vi "Actor Core.vi"(8 "error in":errorcluster, 11 "MWWL Verification":refnum<class "MWWL Verification.lvclass">) -> (0 "error out":errorcluster, 3 "Actor out":refnum<class "Actor.lvclass">)   [LabVIEW 2018, in "MWWL Verification.lvlib" / "MWWL Verification.lvclass"]
doc: "The purpose of this program is to allow an operator to dynamically select a microwave radar water level or bridge clearance (Air Gap) sensor and validate the range measurements by comparing to a series of high precision laser range finders (acquired from Dimetix & Laser Technologies Inc.)."
uses:
  MWWL Verification.lvclass
  C:/Program Files (x86)/National Instruments/LabVIEW 2018/vi.lib/ActorFramework/Actor/Actor.lvclass
  <vilib>/ActorFramework/Actor/Actor.lvclass
  Type Defs/Menu Items.ctl
  Type Defs/DLS Status LEDs.ctl
  Range Controller Actor/Typedefs/Verifier Enum.ctl
  <vilib>/ActorFramework/Actor/Actor.lvclass/Actor.ctl
  <vilib>/ActorFramework/Message Enqueuer/Message Enqueuer.lvclass/Message Enqueuer.ctl
  MWWL Verification.lvclass/MWWL Verification.ctl
  <vilib>/ActorFramework/Message Enqueuer/Init from Existing Queue.vi
  <vilib>/ActorFramework/Message Enqueuer/Enqueue.vi
  <vilib>/ActorFramework/Stop Msg/Stop Msg.lvclass
  C:/Program Files (x86)/National Instruments/LabVIEW 2018/vi.lib/ActorFramework/Message/Message.lvclass
  MWWL Verification Messages/Abort Msg/Abort Msg.lvclass
  <vilib>/ActorFramework/Message Priority Queue/Priority Enqueue.vi
  Actor Monitor/Actor/Monitored Actor.lvclass
  <vilib>/ActorFramework/Message Enqueuer/Message Enqueuer.lvclass
  MWWL Verification Messages/Initialize Reference Range Controller Msg/Initialize Reference Range Controller Msg.lvclass
  MWWL Verification Messages/Disabled Property(Main Controls)_Initialize Msg/Disabled Property(Main Controls)_Initialize Msg.lvclass
  MWWL Verification Messages/Move Target Manually Msg/Move Target Manually Msg.lvclass
  MWWL Verification Messages/Manual or Auto Controller Msg/Manual or Auto Controller Msg.lvclass
  MWWL Verification Messages/Set Desired Range Msg/Set Desired Range Msg.lvclass
  MWWL Verification Messages/Mean Range Values from FP Indicators Msg/Mean Range Values from FP Indicators Msg.lvclass
  MWWL Verification Messages/Disabled Property(Main Controls)_Measure Msg/Disabled Property(Main Controls)_Measure Msg.lvclass
  MWWL Verification Messages/Create Data Entry for Log Msg/Create Data Entry for Log Msg.lvclass
  MWWL Verification Messages/Initialize Datalogger Msg/Initialize Datalogger Msg.lvclass
  MWWL Verification.lvlib
panel:
  in  "Verifier State":T1
  out "Time Series":T2(graph)
  in  "Reference Range Controls":cluster{"FWD":bool, "REV":bool}
  in  "Recording?":bool
  in  "Target Range":dbl(slide) min=0.0 max=30.0 step=0.001 scale=0.0..30.0 scale format="%#.2g"
  in  "Fault?":bool
  in  "Main Controls":T3
  out "Ranges":T5 {"ULS" format="%.3g"; "LASER D" format="%.3g"; "LASER C" format="%.3g"; "LASER B" format="%.3g"; "Microwave" format="%.3g"; "LASER A" format="%.3g"}
  in  "stop signal":bool
  out "Event Log":string
  in  "WebBrowser":refnum<k7>(container)
  # "RANGES (m)"
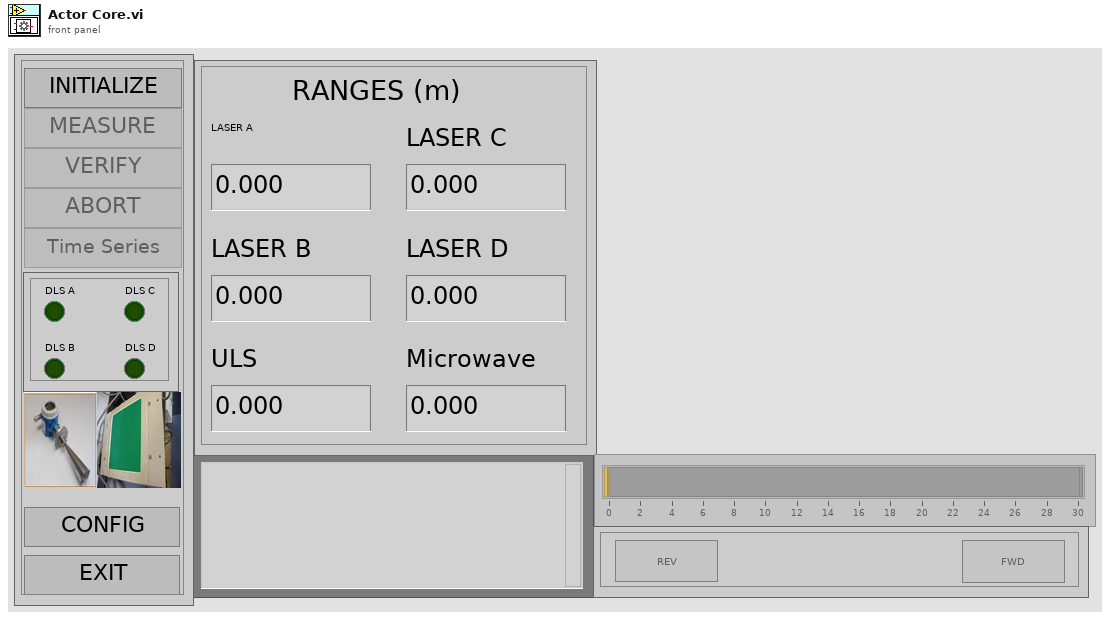
[diagram p1: front panel]
types:
  T1 = typedef "MWWL Verification.lvlib/Verifier Enum.ctl" = enum16{"Idle", "Begin Test", "Check Target Distance", "Move Target", "Save to Disk", "Check Desired Range"}
  T2 = cluster{"NewVal":dbl, "NewVal":dbl, "NewVal":dbl, "NewVal":dbl, "NewVal":dbl, "NewVal":dbl}
  T3 = typedef "MWWL Verification.lvlib/Menu Items.ctl" = cluster{"Initialize":bool, "Measure":bool, "Verify Button":bool, "Abort Button":bool, "Time Series":bool, "ULS Status":T4, "Config Button":bool, "Exit Button":bool}
  T4 = typedef "MWWL Verification.lvlib/DLS Status LEDs.ctl" = cluster{"DLS A":bool, "DLS B":bool, "DLS C":bool, "DLS D":bool}
  T5 = cluster{"LASER A":dbl, "LASER B":dbl, "LASER C":dbl, "LASER D":dbl, "ULS":dbl, "Microwave":dbl}
  T6 = enum8{"Enabled", "Disabled", "Disabled and Grayed Out"}
  T7 = typedef "MWWL Verification.lvlib/ConfigSettings.ctl" = cluster{"Base Path":path, "DNL_Configuration Settings.Ports":cluster{"Ref. Range COM Port":refnum<visa-resource-name>, "MWWL COM Port":refnum<visa-resource-name>, "ULS COM Port":refnum<visa-resource-name>, "Laser A COM Port":refnum<visa-resource-name>, "Laser B COM Port":refnum<visa-resource-name>, "Laser C COM Port":refnum<visa-resource-name>, "Laser D COM Port":refnum<visa-resource-name>, "AirMar COM Port":refnum<visa-resource-name>}, "H3611i":bool}
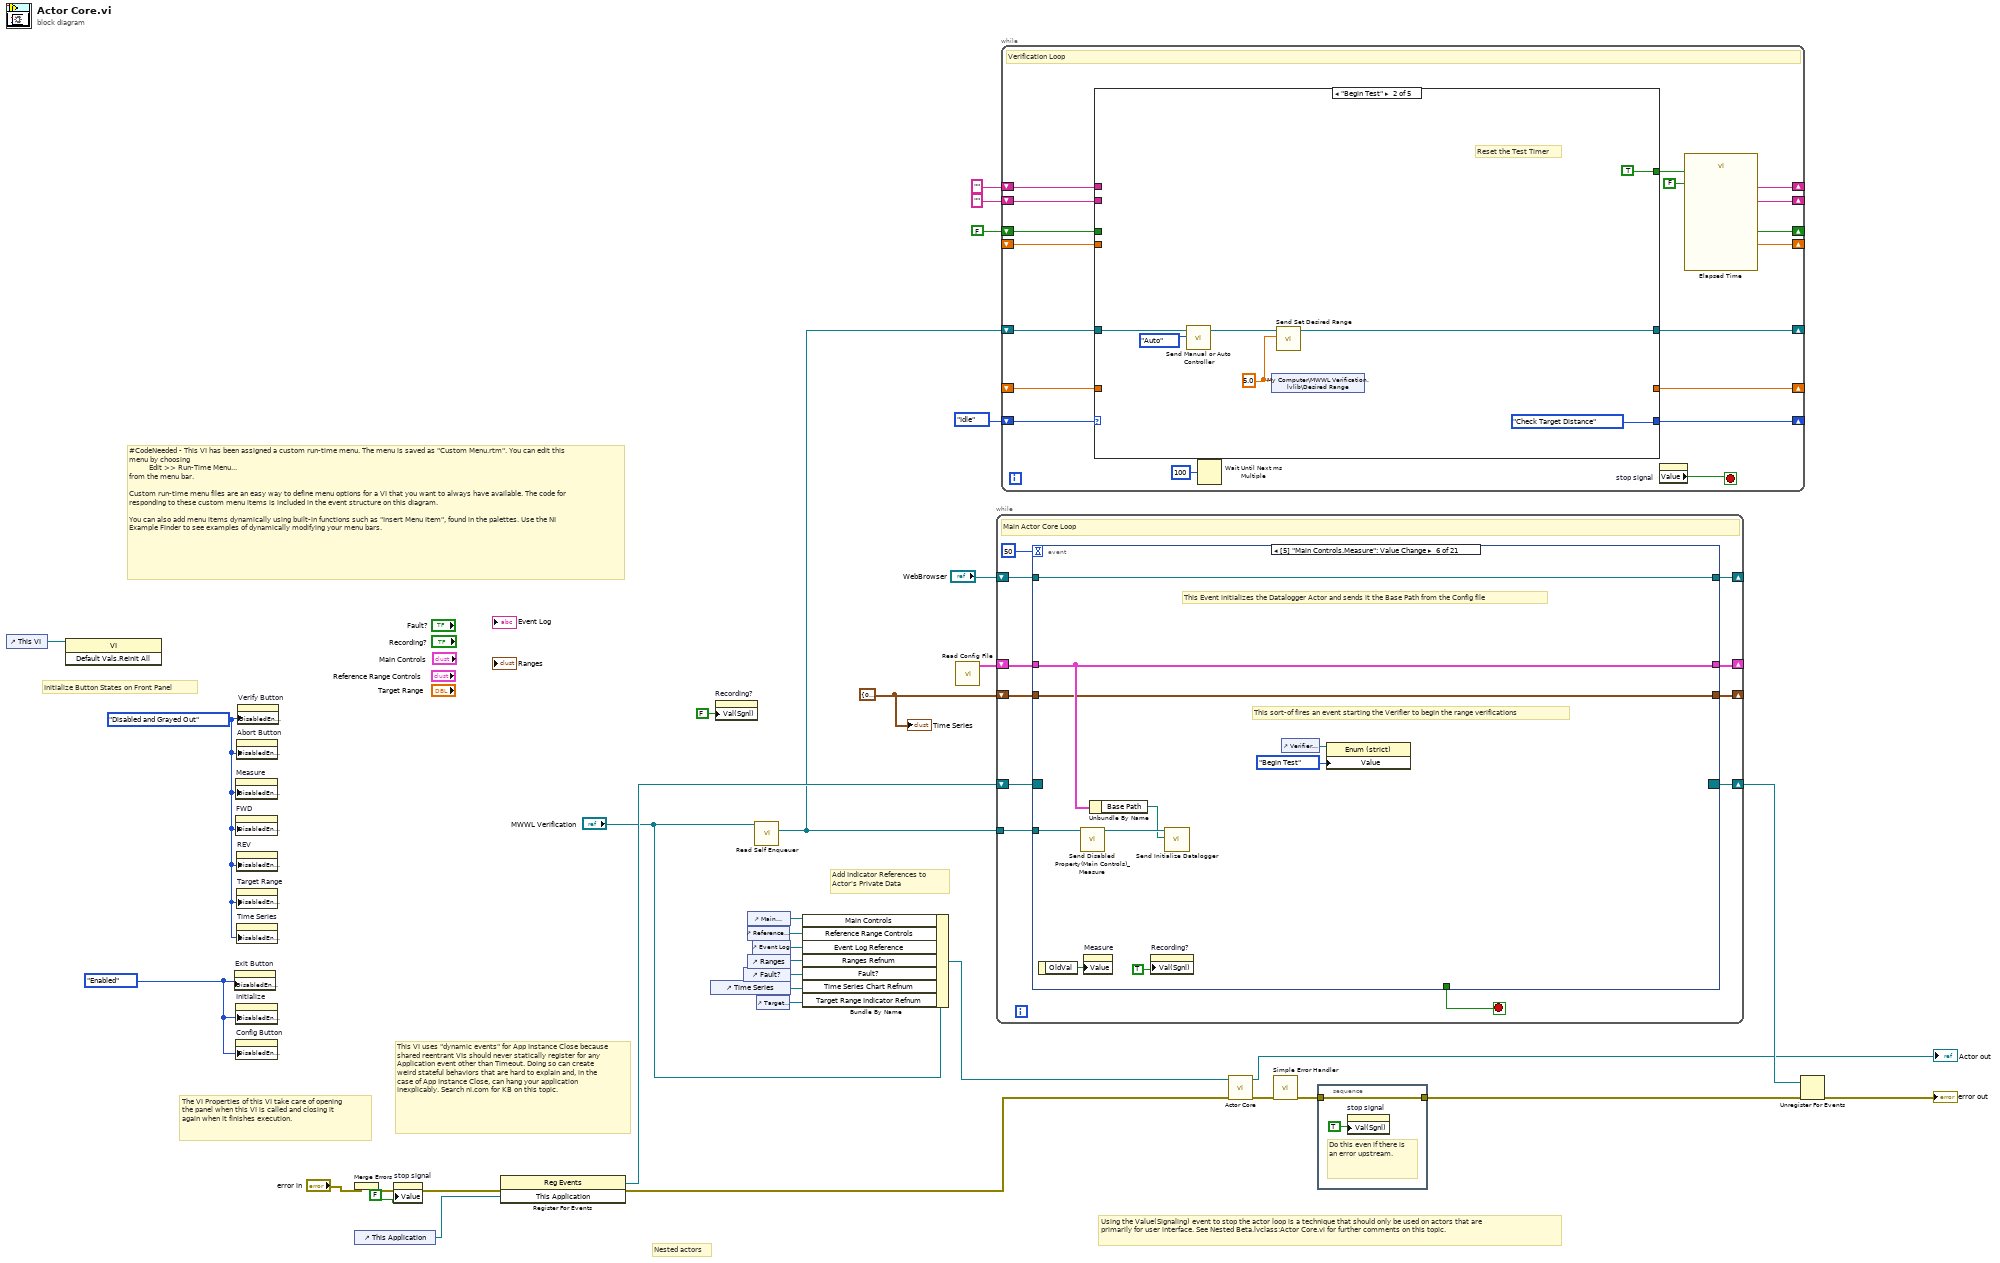
[diagram p0: block diagram]
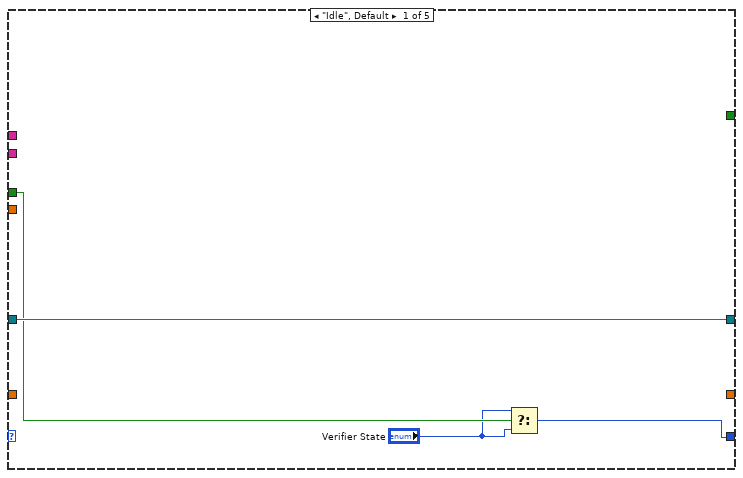
[diagram p2: hidden frame]
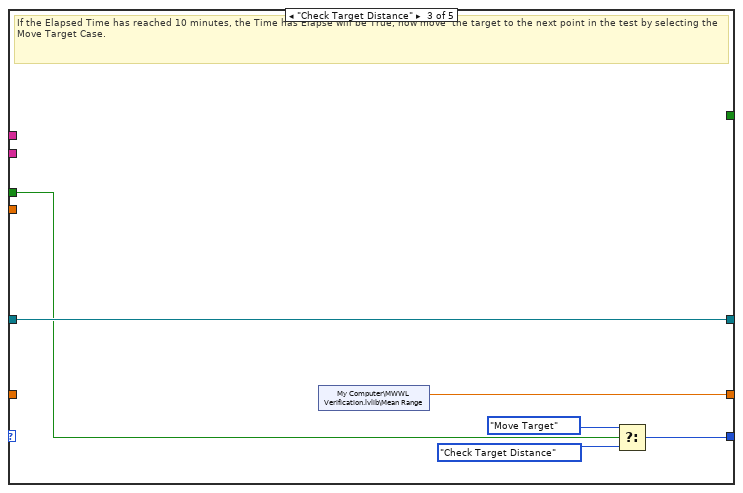
[diagram p3: hidden frame]
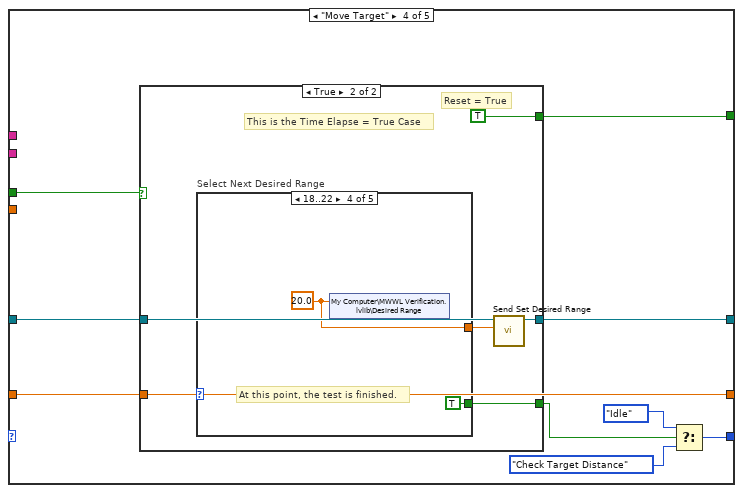
[diagram p4: hidden frame]
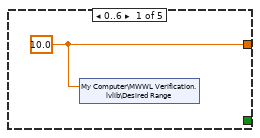
[diagram p6: hidden frame]
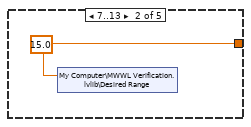
[diagram p7: hidden frame]
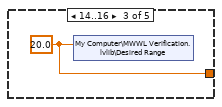
[diagram p8: hidden frame]
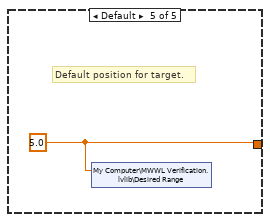
[diagram p9: hidden frame]
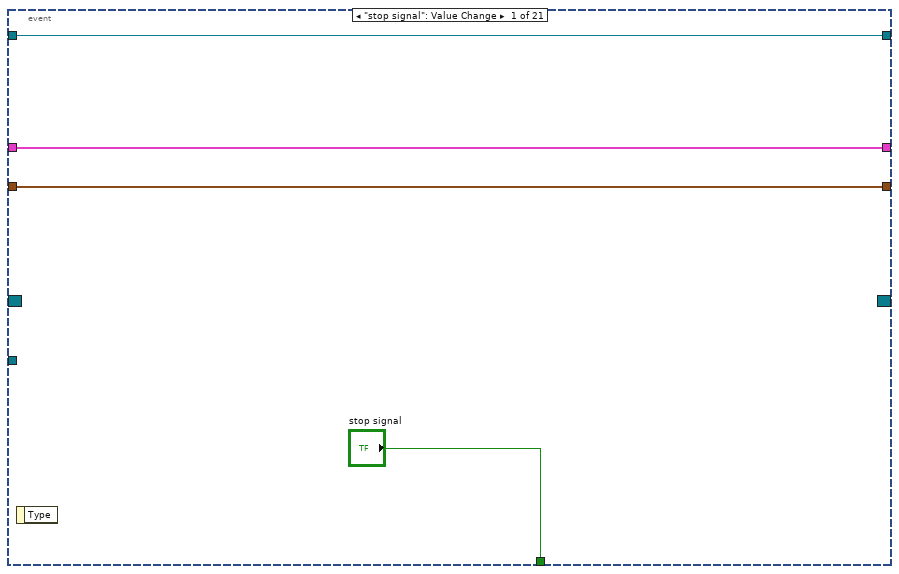
[diagram p11: hidden frame]
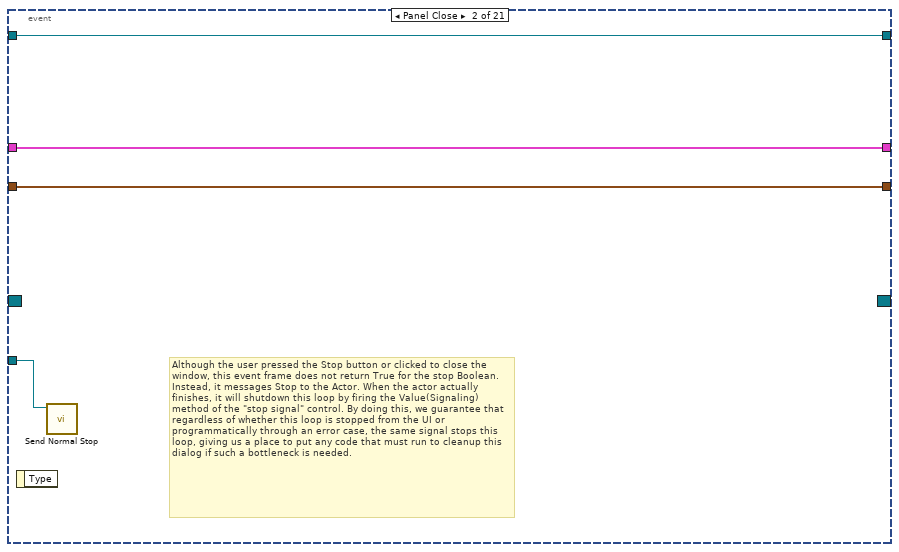
[diagram p12: hidden frame]
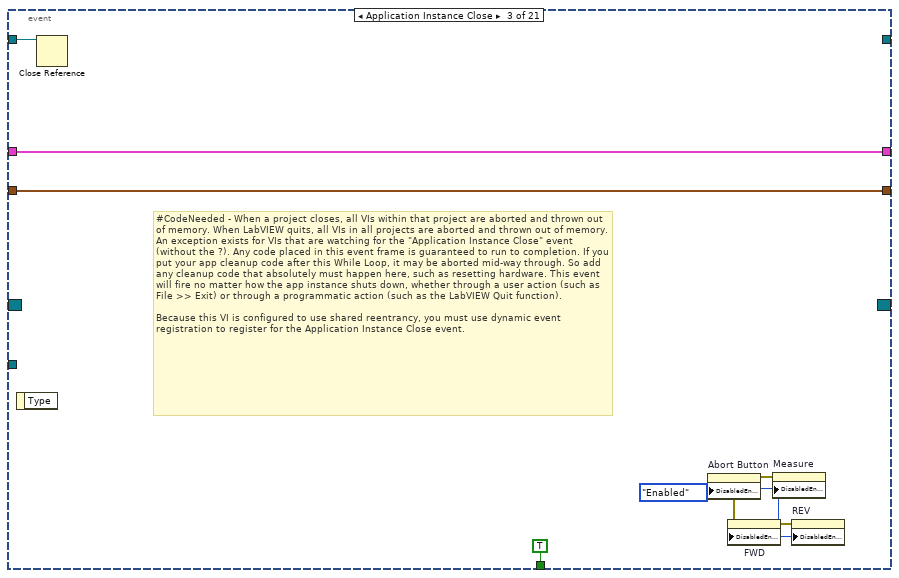
[diagram p13: hidden frame]
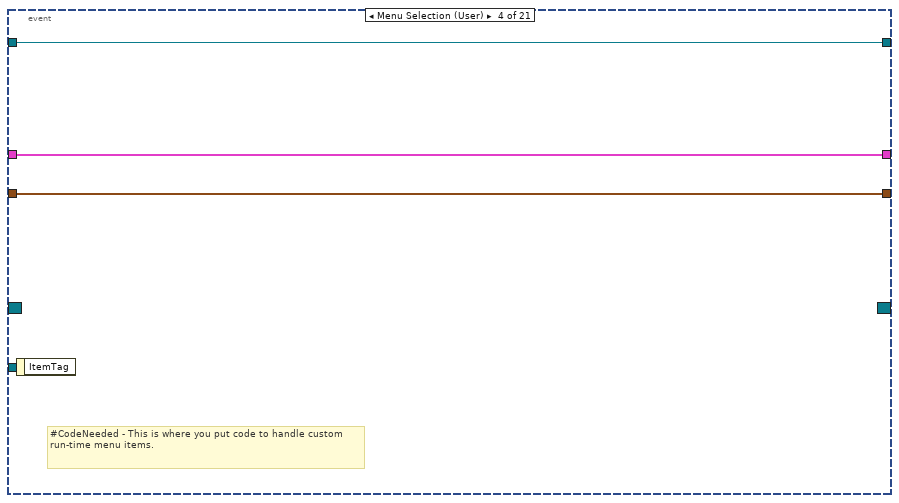
[diagram p14: hidden frame]
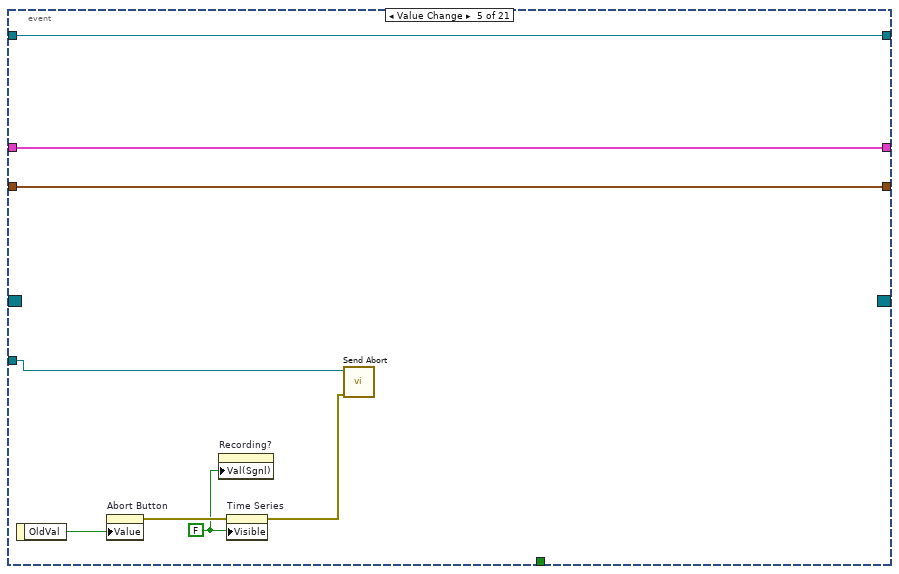
[diagram p15: hidden frame]
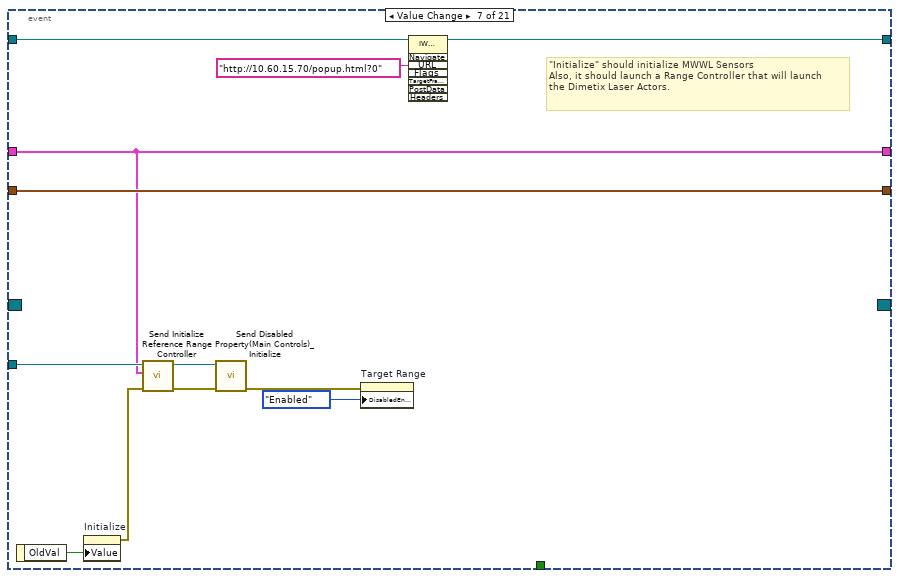
[diagram p16: hidden frame]
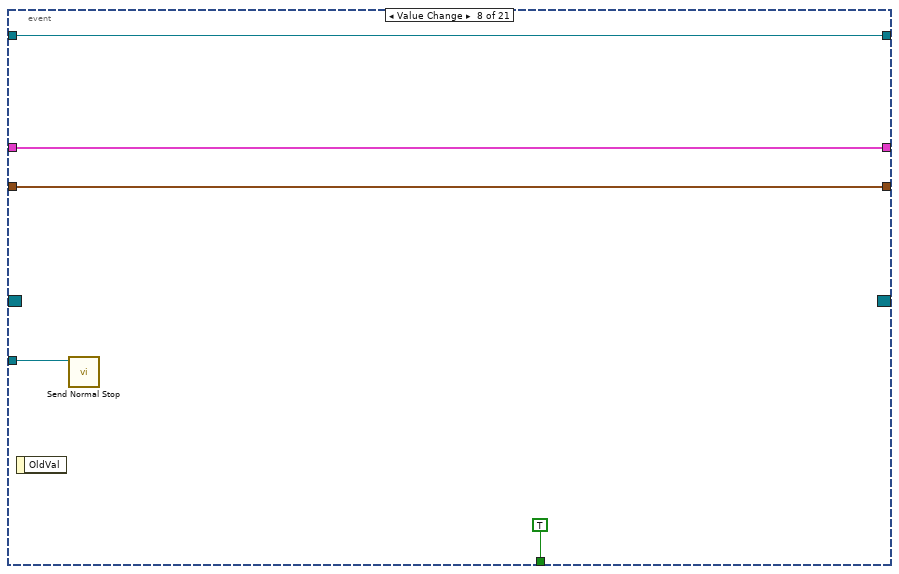
[diagram p17: hidden frame]
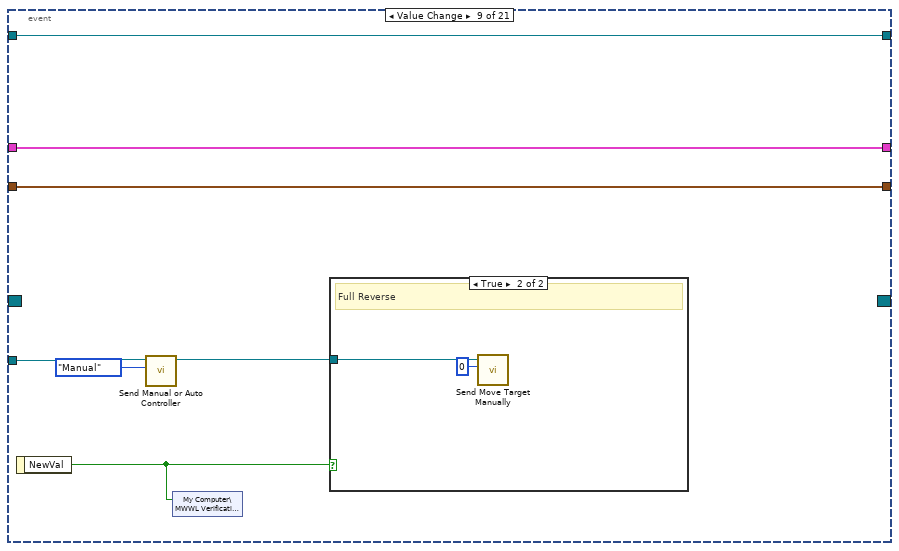
[diagram p18: hidden frame]
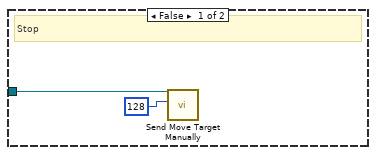
[diagram p19: hidden frame]
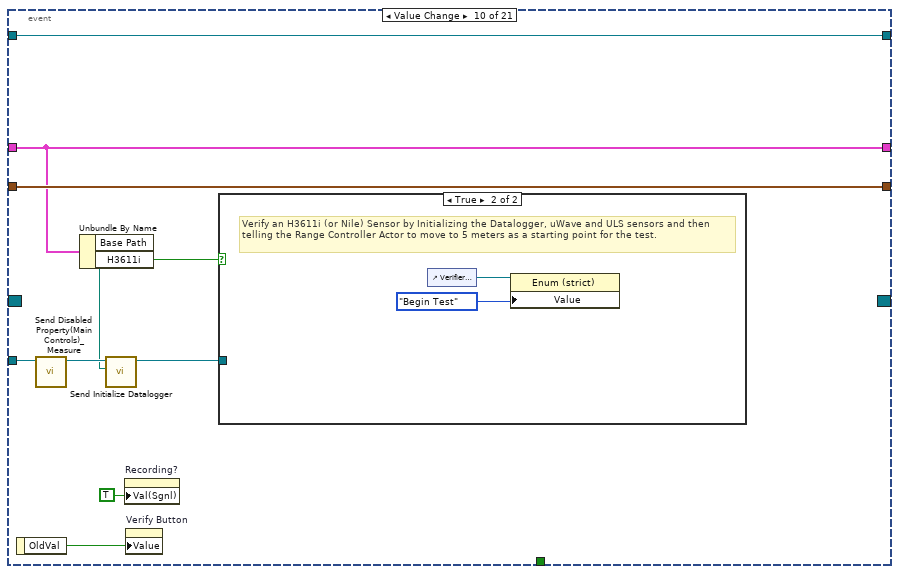
[diagram p20: hidden frame]
diagram:
  w9 = T5 {"LASER A"=0.0, "LASER B"=0.0, "LASER C"=0.0, "LASER D"=0.0, "ULS"=0.0, "Microwave"=0.0} ("Ranges")
  w12 = T6."Disabled and Grayed Out" ("Disabled")
  w11 = T6."Enabled" ("Disabled")
  # "Initialize Button States on Front Panel"
  # "Add Indicator References to \nActor's Private Data"
  # "Nested actors"
  # "#CodeNeeded - This VI has been assigned a custom run-time menu. The menu is saved as \"Custom Menu.rtm\". You can edit this menu by choosing \n          Edit >> Run-Time Menu...\nfrom the menu bar.\n\nCustom run-time menu files are an easy way to define menu options for a VI that you want to always have available. The code for responding to these custom menu items is included in the event structure on this diagram.\n\nYou can also add menu items dynamically using built-in functions such as \"Insert Menu Item\", found in the palettes. Use the NI Example Finder to see examples of dynamically modifying your menu bars."
  # "This VI uses \"dynamic events\" for App Instance Close because shared reentrant VIs should never statically register for any Application event other than Timeout. Doing so can create weird stateful behaviors that are hard to explain and, in the case of App Instance Close, can hang your application inexplicably. Search ni.com for KB on this topic."
  # "The VI Properties of this VI take care of opening the panel when this VI is called and closing it again when it finishes execution."
  # "Using the Value(Signaling) event to stop the actor loop is a technique that should only be used on actors that are primarily for user interface. See Nested Beta.lvclass:Actor Core.vi for further comments on this topic."
  n1 = control-ref of="This VI"() -> (w20:refnum<vi>)
  n2 = invoke class="VI" method="Default Vals.Reinit All"(reference=w20) -> ()  [unwired: 2 in, 3 out]
  n3 = property on="Exit Button" class="Bool"("DisabledEnum"=w11) -> ()  [unwired: 2 in, 2 out]
  n4 = property on="Measure" class="Bool (strict)"("DisabledEnum"=w12) -> ()  [unwired: 2 in, 2 out]
  n5 = property on="FWD" class="Bool (strict)"("DisabledEnum"=w12) -> ()  [unwired: 2 in, 2 out]
  n6 = property on="Initialize" class="Bool (strict)"("DisabledEnum"=w11) -> ()  [unwired: 2 in, 2 out]
  n7 = property on="Config Button" class="Bool (strict)"("DisabledEnum"=w11) -> ()  [unwired: 2 in, 2 out]
  n8 = property on="Abort Button" class="Bool (strict)"("DisabledEnum"=w12) -> ()  [unwired: 2 in, 2 out]
  n9 = property on="REV" class="Bool (strict)"("DisabledEnum"=w12) -> ()  [unwired: 2 in, 2 out]
  n10 = property on="Target Range" class="Slide (strict)"("DisabledEnum"=w12) -> ()  [unwired: 2 in, 2 out]
  n11 = property on="Time Series" class="Bool (strict)"("DisabledEnum"=w12) -> ()  [unwired: 2 in, 2 out]
  n12 = property on="Verify Button" class="Bool (strict)"("DisabledEnum"=w12) -> ()  [unwired: 2 in, 2 out]
  n13 = Merge Errors("error in") -> (w32:errorcluster)
  n14 = control-ref of="This Application"() -> (w3:refnum<vi>)
  n15 = property on="stop signal" class="Bool (strict)"(error in=w32, "Value"=FALSE ("stop")) -> (error out=w26:errorcluster)  [unwired: 1 in, 1 out]
  n16 = register-events(error in=w26, w3) -> (reference out=w29:refnum<event-registration>, error out=w23:errorcluster)  [unwired: 1 in]
  n17 = control-ref of="Time Series"() -> (w10:refnum<vi>)
  n18 = property on="Recording?" class="Bool (strict)"("Val(Sgnl)"=FALSE ("Value (Signaling)")) -> ()  [unwired: 2 in, 2 out]
  n19 = control-ref of="Fault?"() -> (w22:refnum<vi>)
  n20 = control-ref of="Reference Range Controls"() -> (w14:refnum<vi>)
  n21 = control-ref of="Main Controls"() -> (w16:refnum<vi>)
  n22 = control-ref of="Ranges"() -> (w21:refnum<vi>)
  n23 = control-ref of="Event Log"() -> (w34:refnum<vi>)
  n24 = call <vilib>:"Read Self Enqueuer.vi"("Actor"="MWWL Verification") -> ("Self Enqueuer"=w6:refnum<class "Message Enqueuer.lvclass">)  [unwired: 10 in]
  n25 = control-ref of="Target Range"() -> (w15:refnum<vi>)
  n26 = Bundle By Name(cluster="MWWL Verification", "Main Controls"=w16, "Reference Range Controls"=w14, "Event Log Reference"=w34, "Ranges Refnum"=w21, "Fault?"=w22, "Time Series Chart Refnum"=w10, "Target Range Indicator Refnum"=w15) -> (w19:refnum<class "MWWL Verification.lvclass">)
  n27 = call "Read Config File.vi"() -> ("Settings Out"=w25:T7)  [unwired: 10 in, 1 out]
  n28 = while {
    tunnel: w6 -> [w45]
    shift-right: [w42] -> w28
    shift-left: w29 -> [w43]
    shift-right: [w40] -> _
    shift-left: w25 -> [w41]
    shift-right: [w37] -> _
    shift-left: w9 -> [w36]
    shift-right: [w35] -> _
    shift-left: "WebBrowser" -> [w39]
    stop <- w44 stop-if-true
    # "Main Actor Core Loop"
    n29 = event shown="[5] \"Main Controls.Measure\": Value Change" {
      selector: w43 -> [_ _ _ _ _ _ _ _ _ _ _ _ _ _ _ _ _ _ _ _ _]
      dyn-events: [_ _ _ _ _ _ _ _ _ _ _ _ _ _ _ _ _ _ _ _ _] -> w42
      timeout: 50 -> [_ _ _ _ _ _ _ _ _ _ _ _ _ _ _ _ _ _ _ _ _]
      tunnel: w45 -> [_ w53 _ _ w71 w81 w91 w99 w105 w114 w126 w139 _ w153 _ w169 w187 w205 w223 w241 w252]
      tunnel: ["stop signal" _ TRUE ("stop signal") _ _ _ _ TRUE ("stop signal") _ _ _ _ _ _ _ _ _ _ _ _ _] -> w44
      tunnel: w41 -> [w48 w52 w61 w64 w72 w79 w83 w97 w106 w115 w129 w140 w146 w154 w162 w170 w188 w206 w224 w242 w253]
      tunnel: [w48 w52 w61 w64 w72 w79 w83 w97 w106 w115 w129 w140 w146 w154 w161 w170 w188 w206 w224 w242 w253] -> w40
      tunnel: w39 -> [w46 w50 w56 w62 w65 w75 w94 w95 w100 w118 w123 w134 w141 w149 w159 w164 w182 w200 w219 w236 w247]
      tunnel: w36 -> [w47 w51 w55 w63 w67 w76 w85 w96 w101 w119 w124 w135 w144 w150 w160 w167 w185 w203 w218 w238 w249]
      tunnel: [w47 w51 w55 w63 w67 w76 w85 w96 w101 w119 w124 w135 w144 w150 w160 w166 w183 w202 w220 w237 w248] -> w37
      tunnel: [w46 w50 _ w62 w65 w75 w84 w95 w100 w118 w123 w134 w141 w149 w159 w164 w182 w200 w219 w236 w247] -> w35
      event "stop signal": Value Change {
        n30 = event-data() -> ()  [unwired: 1 in, 1 out]
      }
      event Panel Close {
        # "Although the user pressed the Stop button or clicked to close the window, this event frame does not return True for the stop Boolean. Instead, it messages Stop to the Actor. When the actor actually finishes, it will shutdown this loop by firing the Value(Signaling) method of the \"stop signal\" control. By doing this, we guarantee that regardless of whether this loop is stopped from the UI or programmatically through an error case, the same signal stops this loop, giving us a place to put any code that must run to cleanup this dialog if such a bottleneck is needed."
        n31 = event-data() -> ()  [unwired: 1 in, 1 out]
        n32 = call <vilib>:"Send Normal Stop.vi"("Message Enqueuer"=w53) -> ()  [unwired: 10 in, 1 out]
      }
      event Application Instance Close {
        w58 = T6."Enabled" ("Disabled")
        # "#CodeNeeded - When a project closes, all VIs within that project are aborted and thrown out of memory. When LabVIEW quits, all VIs in all projects are aborted and thrown out of memory. An exception exists for VIs that are watching for the \"Application Instance Close\" event (without the ?). Any code placed in this event frame is guaranteed to run to completion. If you put your app cleanup code after this While Loop, it may be aborted mid-way through. So add any cleanup code that absolutely must happen here, such as resetting hardware. This event will fire no matter how the app instance shuts down, whether through a user action (such as File >> Exit) or through a programmatic action (such as the LabVIEW Quit function).\n\nBecause this VI is configured to use shared reentrancy, you must use dynamic event registration to register for the Application Instance Close event."
        n33 = event-data() -> ()  [unwired: 1 in, 1 out]
        n34 = Close Reference(reference=w56) -> ()  [unwired: 1 in, 1 out]
        n35 = property on="Abort Button" class="Bool (strict)"("DisabledEnum"=w58) -> (error out=w57:errorcluster)  [unwired: 2 in, 1 out]
        n36 = property on="Measure" class="Bool (strict)"(error in=w57, "DisabledEnum"=w58) -> (error out=w59:errorcluster)  [unwired: 1 in, 1 out]
        n37 = property on="FWD" class="Bool (strict)"(error in=w59, "DisabledEnum"=w58) -> (error out=w60:errorcluster)  [unwired: 1 in, 1 out]
        n38 = property on="REV" class="Bool (strict)"(error in=w60, "DisabledEnum"=w58) -> ()  [unwired: 1 in, 2 out]
      }
      event Menu Selection (User) {
        # "#CodeNeeded - This is where you put code to handle custom run-time menu items."
        n39 = event-data() -> ()  [unwired: 1 in, 1 out]
      }
      event Value Change {
        w66 = FALSE ("Visible")
        n40 = event-data() -> ("OldVal"=w70:bool)  [unwired: 1 in]
        n41 = property on="Abort Button" class="Bool (strict)"("Value"=w70) -> (error out=w69:errorcluster)  [unwired: 2 in, 1 out]
        n42 = property on="Recording?" class="Bool (strict)"("Val(Sgnl)"=w66) -> ()  [unwired: 2 in, 2 out]
        n43 = property on="Time Series" class="WFChart (strict)"(error in=w69, "Visible"=w66) -> (error out=w68:errorcluster)  [unwired: 1 in, 1 out]
        n44 = call "Send Abort.vi"("error in (no error)"=w68, "Message Enqueuer in"=w71) -> ()  [unwired: 8 in, 2 out]
      }
      event Value Change {
        # "This sort-of fires an event starting the Verifier to begin the range verifications"
        # "This Event initializes the Datalogger Actor and sends it the Base Path from the Config file"
        n45 = event-data() -> ("OldVal"=w82:bool)  [unwired: 1 in]
        n46 = call "Send Disabled Property(Main Controls)_Measure.vi"("Message Enqueuer in"=w81) -> ("Message Enqueuer out"=w80:refnum<class "Message Enqueuer.lvclass">)  [unwired: 9 in, 1 out]
        n47 = property on="Measure" class="Bool (strict)"("Value"=w82) -> ()  [unwired: 2 in, 2 out]
        n48 = Unbundle By Name(w79) -> ("Base Path"=w78:path)
        n49 = property on="Recording?" class="Bool (strict)"("Val(Sgnl)"=TRUE ("Value (Signaling)")) -> ()  [unwired: 2 in, 2 out]
        n50 = call "Send Initialize Datalogger.vi"("Base File Path"=w78, "Message Enqueuer in"=w80) -> ()  [unwired: 8 in, 2 out]
        n51 = control-ref of="Verifier State"() -> (w74:refnum<vi>)
        n52 = property class="Enum (strict)"(reference=w74, "Value"=Verifier_Enum."Begin Test" ("Verifier State")) -> ()  [unwired: 1 in, 2 out]
      }
      event Value Change {
        # "\"Initialize\" should initialize MWWL Sensors\nAlso, it should launch a Range Controller that will launch\nthe Dimetix Laser Actors."
        n53 = event-data() -> ("OldVal"=w89:bool)  [unwired: 1 in]
        n54 = property on="Initialize" class="Bool (strict)"("Value"=w89) -> (error out=w88:errorcluster)  [unwired: 2 in, 1 out]
        n55 = call "Send Initialize Reference Range Controller.vi"("error in (no error)"=w88, "Settings"=w83, "Message Enqueuer in"=w91) -> ("error out"=w90:errorcluster, "Message Enqueuer out"=w92:refnum<class "Message Enqueuer.lvclass">)  [unwired: 7 in]
        n56 = call "Send Disabled Property(Main Controls)_Initialize.vi"("error in (no error)"=w90, "Message Enqueuer in"=w92) -> ("error out"=w86:errorcluster)  [unwired: 8 in, 1 out]
        n57 = property on="Target Range" class="Slide (strict)"(error in=w86, "DisabledEnum"=T6."Enabled" ("Disabled")) -> ()  [unwired: 1 in, 2 out]
        n58 = invoke class="IWebBrowser2" method="Navigate"(reference=w94, "URL"="http://10.60.15.70/popup.html?0") -> (reference out=w84:refnum<k7>)  [unwired: 6 in, 7 out]
      }
      event Value Change {
        n59 = event-data() -> ()  [unwired: 1 in, 1 out]
        n60 = call <vilib>:"Send Normal Stop.vi"("Message Enqueuer"=w99) -> ()  [unwired: 10 in, 1 out]
      }
      event "Reference Range Controls.FWD": Value Change {
        n61 = event-data() -> ("NewVal"=w102:bool)  [unwired: 1 in]
        n62 = call "Send Manual or Auto Controller.vi"("Controller State"=enum16{"Manual", "Auto"}."Manual", "Message Enqueuer in"=w105) -> ("Message Enqueuer out"=w103:refnum<class "Message Enqueuer.lvclass">)  [unwired: 8 in, 1 out]
        n63 = shared-variable "My Computer\\MWWL Verification.lvlib\\FWD"(w102) -> ()  [unwired: 1 in, 1 out]
        n64 = case shown="True" w102 {
          tunnel: w103 -> [w107 w110]
          frame False {
            # "Stop"
            n65 = call "Send Move Target Manually.vi"("Target Speed & Direction"=i16 128, "Message Enqueuer in"=w107) -> ()  [unwired: 8 in, 2 out]
          }
          frame True {
            # "Full Reverse"
            n66 = call "Send Move Target Manually.vi"("Target Speed & Direction"=i16 0, "Message Enqueuer in"=w110) -> ()  [unwired: 8 in, 2 out]
          }
        }
      }
      event Value Change {
        n67 = event-data() -> ("OldVal"=w120:bool)  [unwired: 1 in]
        n68 = call "Send Disabled Property(Main Controls)_Measure.vi"("Message Enqueuer in"=w114) -> ("Message Enqueuer out"=w117:refnum<class "Message Enqueuer.lvclass">)  [unwired: 9 in, 1 out]
        n69 = Unbundle By Name(w115) -> ("Base Path"=w116:path, "H3611i"=w112:bool)
        n70 = call "Send Initialize Datalogger.vi"("Base File Path"=w116, "Message Enqueuer in"=w117) -> ("Message Enqueuer out"=w111:refnum<class "Message Enqueuer.lvclass">)  [unwired: 8 in, 1 out]
        n71 = property on="Recording?" class="Bool (strict)"("Val(Sgnl)"=TRUE ("Value (Signaling)")) -> ()  [unwired: 2 in, 2 out]
        n72 = property on="Verify Button" class="Bool (strict)"("Value"=w120) -> ()  [unwired: 2 in, 2 out]
        n73 = case shown="True" w112 {
          tunnel: w111 -> [_ _]
          frame False {
          }
          frame True {
            # "Verify an H3611i (or Nile) Sensor by Initializing the Datalogger, uWave and ULS sensors and then telling the Range Controller Actor to move to 5 meters as a starting point for the test."
            n74 = control-ref of="Verifier State"() -> (w122:refnum<vi>)
            n75 = property class="Enum (strict)"(reference=w122, "Value"=Verifier_Enum."Begin Test" ("Verifier State")) -> ()  [unwired: 1 in, 2 out]
          }
        }
      }
      event "Reference Range Controls.REV": Value Change {
        n76 = event-data() -> ("NewVal"=w125:bool)  [unwired: 1 in]
        n77 = shared-variable "My Computer\\MWWL Verification.lvlib\\REV"(w125) -> ()  [unwired: 1 in, 1 out]
        n78 = call "Send Manual or Auto Controller.vi"("Controller State"=enum16{"Manual", "Auto"}."Manual", "Message Enqueuer in"=w126) -> ("Message Enqueuer out"=w128:refnum<class "Message Enqueuer.lvclass">)  [unwired: 8 in, 1 out]
        n79 = case shown="True" w125 {
          tunnel: w128 -> [w130 w133]
          frame False {
            # "Stop"
            n80 = call "Send Move Target Manually.vi"("Target Speed & Direction"=i16 128, "Message Enqueuer in"=w130) -> ()  [unwired: 8 in, 2 out]
          }
          frame True {
            # "Full Reverse"
            n81 = call "Send Move Target Manually.vi"("Target Speed & Direction"=i16 255, "Message Enqueuer in"=w133) -> ()  [unwired: 8 in, 2 out]
          }
        }
      }
      event "Target Range": Value Change {
        n82 = event-data() -> ("NewVal"=w136:dbl)  [unwired: 1 in]
        n83 = call "Send Manual or Auto Controller.vi"("Controller State"=enum16{"Manual", "Auto"}."Auto", "Message Enqueuer in"=w139) -> ("Message Enqueuer out"=w137:refnum<class "Message Enqueuer.lvclass">)  [unwired: 8 in, 1 out]
        n84 = shared-variable "My Computer\\MWWL Verification.lvlib\\Desired Range"(w136) -> ()  [unwired: 1 in, 1 out]
        n85 = call "Send Set Desired Range.vi"("Desired Range"=w136, "Message Enqueuer in"=w137) -> ()  [unwired: 8 in, 2 out]
      }
      event Value Change {
        n86 = event-data() -> ("OldVal"=w145:bool)  [unwired: 1 in]
        n87 = property on="Time Series" class="Bool (strict)"("Value"=w145) -> ()  [unwired: 2 in, 2 out]
        n88 = control-ref of="Time Series"() -> (w148:refnum<vi>)
        n89 = property class="WFChart (strict)"(reference=w148) -> (reference out=w147:refnum<vi>, "Visible"=w142:bool)  [unwired: 1 in, 1 out]
        n90 = Not(x=w142) -> (.not. x?=w143:bool)
        n91 = property class="WFChart (strict)"(reference=w147, "Visible"=w143) -> ()  [unwired: 1 in, 2 out]
        n92 = property on="WebBrowser" class="AXCont"("Visible"=w142) -> ()  [unwired: 2 in, 2 out]
      }
      event Timeout {
        n93 = event-data() -> ()  [unwired: 1 in, 1 out]
        n94 = call "Send Mean Range Values from FP Indicators.vi"("Message Enqueuer in"=w153) -> ()  [unwired: 9 in, 2 out]
        n95 = control-ref of="FWD"() -> (w157:refnum<vi>)
        n96 = shared-variable "My Computer\\MWWL Verification.lvlib\\FWD"() -> (w158:bool)  [unwired: 1 in, 1 out]
        n97 = shared-variable "My Computer\\MWWL Verification.lvlib\\REV"() -> (w155:bool)  [unwired: 1 in, 1 out]
        n98 = control-ref of="REV"() -> (w156:refnum<vi>)
        n99 = control-ref of="Target Range"() -> (w152:refnum<vi>)
        n100 = shared-variable "My Computer\\MWWL Verification.lvlib\\Desired Range"() -> (w151:dbl)  [unwired: 1 in, 1 out]
        n101 = property class="Bool (strict)"(reference=w157, "Value"=w158) -> ()  [unwired: 1 in, 2 out]
        n102 = property class="Bool (strict)"(reference=w156, "Value"=w155) -> ()  [unwired: 1 in, 2 out]
        n103 = property class="Slide (strict)"(reference=w152, "Value"=w151) -> ()  [unwired: 1 in, 2 out]
      }
      event Value Change {
        n104 = event-data() -> ("OldVal"=w163:bool)  [unwired: 1 in]
        n105 = property on="Config Button" class="Bool (strict)"("Value"=w163) -> ()  [unwired: 2 in, 2 out]
        n106 = call "Write Config File.vi"("Settings"=w162) -> ("Settings Out"=w161:T7)  [unwired: 9 in, 1 out]
      }
      event "Ranges.LASER A": Value Change {
        n107 = event-data() -> ("NewVal"=w165:dbl)  [unwired: 1 in]
        n108 = property on="Recording?" class="Bool (strict)"() -> ("Value"=w168:bool)  [unwired: 2 in, 2 out]
        n109 = Bundle By Name(cluster=w167, "LASER A"=w165) -> (w166:T5)
        n110 = case shown="True" w168 {
          tunnel: w169 -> [_ w173]
          tunnel: w165 -> [_ w172]
          frame False {
          }
          frame True {
            n111 = property on="DLS A" class="Bool (strict)"() -> ("Value"=w171:bool)  [unwired: 2 in, 2 out]
            n112 = case shown="True" w171 {
              tunnel: w173 -> [w175 w181]
              tunnel: w172 -> [w174 _]
              frame False {
                # "Laser A"
                n113 = call "Send Create Data Entry for Log.vi"("Units"="m", "Sensor Name"="A", "Data In"=w174, "Message Enqueuer in"=w175) -> ()  [unwired: 6 in, 2 out]
              }
              frame True {
                # "Laser A"
                n114 = call "Send Create Data Entry for Log.vi"("Units"="m", "Sensor Name"="A", "Data In"=0.0, "Message Enqueuer in"=w181) -> ()  [unwired: 6 in, 2 out]
              }
            }
          }
        }
        n115 = property on="Time Series" class="WFChart (strict)"("Value"=w166) -> ()  [unwired: 2 in, 2 out]
      }
      event "Ranges.LASER B": Value Change {
        n116 = event-data() -> ("NewVal"=w184:dbl)  [unwired: 1 in]
        n117 = property on="Recording?" class="Bool (strict)"() -> ("Value"=w186:bool)  [unwired: 2 in, 2 out]
        n118 = Bundle By Name(cluster=w185, "LASER B"=w184) -> (w183:T5)
        n119 = case shown="True" w186 {
          tunnel: w187 -> [_ w191]
          tunnel: w184 -> [_ w190]
          frame False {
          }
          frame True {
            n120 = property on="DLS B" class="Bool (strict)"() -> ("Value"=w189:bool)  [unwired: 2 in, 2 out]
            n121 = case shown="False" w189 {
              tunnel: w191 -> [w195 w199]
              tunnel: w190 -> [_ w198]
              frame True {
                # "If sensor is in \nerror state, log\na zero."
                # "Laser B"
                n122 = call "Send Create Data Entry for Log.vi"("Units"="m", "Sensor Name"="B", "Data In"=0.0, "Message Enqueuer in"=w195) -> ()  [unwired: 6 in, 2 out]
              }
              frame False {
                # "Sensor not in\nerror state. Log\nValue."
                # "Laser B"
                n123 = call "Send Create Data Entry for Log.vi"("Units"="m", "Sensor Name"="B", "Data In"=w198, "Message Enqueuer in"=w199) -> ()  [unwired: 6 in, 2 out]
              }
            }
          }
        }
        n124 = property on="Time Series" class="WFChart (strict)"("Value"=w183) -> ()  [unwired: 2 in, 2 out]
      }
      event "Ranges.LASER C": Value Change {
        n125 = event-data() -> ("NewVal"=w201:dbl)  [unwired: 1 in]
        n126 = property on="Recording?" class="Bool (strict)"() -> ("Value"=w204:bool)  [unwired: 2 in, 2 out]
        n127 = Bundle By Name(cluster=w203, "LASER C"=w201) -> (w202:T5)
        n128 = case shown="True" w204 {
          tunnel: w205 -> [_ w209]
          tunnel: w201 -> [_ w208]
          frame False {
          }
          frame True {
            n129 = property on="DLS C" class="Bool (strict)"() -> ("Value"=w207:bool)  [unwired: 2 in, 2 out]
            n130 = case shown="False" w207 {
              tunnel: w209 -> [w213 w215]
              tunnel: w208 -> [w212 _]
              frame False {
                # "Laser C"
                n131 = call "Send Create Data Entry for Log.vi"("Units"="m", "Sensor Name"="C", "Data In"=w212, "Message Enqueuer in"=w213) -> ()  [unwired: 6 in, 2 out]
              }
              frame True {
                # "Laser C"
                n132 = call "Send Create Data Entry for Log.vi"("Units"="m", "Sensor Name"="C", "Data In"=0.0, "Message Enqueuer in"=w215) -> ()  [unwired: 6 in, 2 out]
              }
            }
          }
        }
        n133 = property on="Time Series" class="WFChart (strict)"("Value"=w202) -> ()  [unwired: 2 in, 2 out]
      }
      event "Ranges.LASER D": Value Change {
        # "There may be a more effective way to log the data."
        n134 = event-data() -> ("NewVal"=w221:dbl)  [unwired: 1 in]
        n135 = Bundle By Name(cluster=w218, "LASER D"=w221) -> (w220:T5)
        n136 = property on="Recording?" class="Bool (strict)"() -> ("Value"=w222:bool)  [unwired: 2 in, 2 out]
        n137 = case shown="True" w222 {
          tunnel: w223 -> [_ w227]
          tunnel: w221 -> [_ w226]
          frame False {
          }
          frame True {
            n138 = property on="DLS D" class="Bool (strict)"() -> ("Value"=w225:bool)  [unwired: 2 in, 2 out]
            n139 = case shown="True" w225 {
              tunnel: w227 -> [w229 w235]
              tunnel: w226 -> [w228 _]
              frame False {
                # "Laser D"
                n140 = call "Send Create Data Entry for Log.vi"("Units"="m", "Sensor Name"="D", "Data In"=w228, "Message Enqueuer in"=w229) -> ()  [unwired: 6 in, 2 out]
              }
              frame True {
                # "Laser D"
                n141 = call "Send Create Data Entry for Log.vi"("Units"="m", "Sensor Name"="D", "Data In"=0.0, "Message Enqueuer in"=w235) -> ()  [unwired: 6 in, 2 out]
              }
            }
          }
        }
        n142 = property on="Time Series" class="WFChart (strict)"("Value"=w220) -> ()  [unwired: 2 in, 2 out]
      }
      event "Ranges.ULS": Value Change {
        n143 = event-data() -> ("NewVal"=w239:dbl)  [unwired: 1 in]
        n144 = property on="Recording?" class="Bool (strict)"() -> ("Value"=w240:bool)  [unwired: 2 in, 2 out]
        n145 = Bundle By Name(cluster=w238, "ULS"=w239) -> (w237:T5)
        n146 = case shown="True" w240 {
          tunnel: w241 -> [_ w246]
          tunnel: w239 -> [_ w245]
          frame False {
          }
          frame True {
            # "ULS"
            n147 = call "Send Create Data Entry for Log.vi"("Units"="m", "Sensor Name"="ULS", "Data In"=w245, "Message Enqueuer in"=w246) -> ()  [unwired: 6 in, 2 out]
          }
        }
        n148 = property on="Time Series" class="WFChart (strict)"("Value"=w237) -> ()  [unwired: 2 in, 2 out]
      }
      event "Ranges.Microwave": Value Change {
        n149 = event-data() -> ("NewVal"=w250:dbl)  [unwired: 1 in]
        n150 = property on="Recording?" class="Bool (strict)"() -> ("Value"=w251:bool)  [unwired: 2 in, 2 out]
        n151 = Bundle By Name(cluster=w249, "Microwave"=w250) -> (w248:T5)
        n152 = case shown="True" w251 {
          tunnel: w252 -> [_ w257]
          tunnel: w250 -> [_ w256]
          frame False {
          }
          frame True {
            # "uWave"
            n153 = call "Send Create Data Entry for Log.vi"("Units"="m", "Sensor Name"="uW", "Data In"=w256, "Message Enqueuer in"=w257) -> ()  [unwired: 6 in, 2 out]
          }
        }
        n154 = property on="Time Series" class="WFChart (strict)"("Value"=w248) -> ()  [unwired: 2 in, 2 out]
      }
    }
  }
  n155 = while {
    shift-right: [w272] -> _
    shift-left: w6 -> [w273]
    shift-right: [w270] -> _
    shift-left: FALSE ("Time has Elapsed") -> [w269]
    shift-right: [w267] -> _
    shift-left: "" ("Start Time Text") -> [w266]
    shift-right: [w265] -> _
    shift-left: _ -> [w264]
    shift-right: [w263] -> _
    shift-left: _ -> [w262]
    shift-right: [w260] -> _
    shift-left: Verifier_Enum."Idle" ("Verifier State") -> [w261]
    shift-right: [w259] -> _
    shift-left: "" ("Elapsed Time Text") -> [w258]
    stop <- w275 stop-if-true
    # "Verification Loop"
    n156 = case shown="\"Begin Test\"" w261 {
      tunnel: [w277 Verifier_Enum."Check Target Distance" ("Verifier State") w290 w296 _] -> w260
      tunnel: w273 -> [w279 w283 w292 w301 w315]
      tunnel: [w279 w282 w292 w300 w315] -> w272
      tunnel: [_ _ w287 w297 _] -> w265
      tunnel: [_ TRUE ("Reset") _ w298 _] -> w271
      tunnel: w269 -> [w278 _ w291 w299 _]
      tunnel: w266 -> [_ _ _ _ _]
      tunnel: w264 -> [_ _ _ w297 _]
      tunnel: w262 -> [_ _ _ _ _]
      tunnel: w258 -> [_ _ _ _ _]
      frame "Idle", Default {
        n157 = Select(t="Verifier State", s=w278, f="Verifier State") -> (s? t:f=w277:T1)
      }
      frame "Begin Test" {
        w284 = 5.0 ("Desired Range")
        # "Reset the Test Timer"
        n158 = call "Send Manual or Auto Controller.vi"("Controller State"=enum16{"Manual", "Auto"}."Auto", "Message Enqueuer in"=w283) -> ("Message Enqueuer out"=w286:refnum<class "Message Enqueuer.lvclass">)  [unwired: 8 in, 1 out]
        n159 = shared-variable "My Computer\\MWWL Verification.lvlib\\Desired Range"(w284) -> ()  [unwired: 1 in, 1 out]
        n160 = call "Send Set Desired Range.vi"("Desired Range"=w284, "Message Enqueuer in"=w286) -> ("Message Enqueuer out"=w282:refnum<class "Message Enqueuer.lvclass">)  [unwired: 8 in, 1 out]
      }
      frame "Check Target Distance" {
        # "If the Elapsed Time has reached 10 minutes, the Time has Elapse will be True, now move  the target to the next point in the test by selecting the Move Target Case."
        n161 = shared-variable "My Computer\\MWWL Verification.lvlib\\Mean Range"() -> (w287:dbl)  [unwired: 1 in, 1 out]
        n162 = Select(t=Verifier_Enum."Move Target" ("Verifier State"), s=w291, f=Verifier_Enum."Check Target Distance" ("Verifier State")) -> (s? t:f=w290:T1)
      }
      frame "Move Target" {
        n163 = case shown="True" w299 {
          tunnel: w301 -> [w302 w308]
          tunnel: [w302 w307] -> w300
          tunnel: [_ TRUE] -> w298
          tunnel: w297 -> [_ w304]
          tunnel: [_ w303] -> w295
          frame False {
          }
          frame True {
            # "This is the Time Elapse = True Case"
            # "Reset = True"
            n164 = case "Select Next Desired Range" shown="18..22" w304 {
              tunnel: [w309 w310 w311 w313 w314] -> w306
              tunnel: [_ _ _ TRUE _] -> w303
              frame 0..6 {
                w309 = 10.0 ("Desired Range")
                n165 = shared-variable "My Computer\\MWWL Verification.lvlib\\Desired Range"(w309) -> ()  [unwired: 1 in, 1 out]
              }
              frame 7..13 {
                w310 = 15.0 ("Desired Range")
                n166 = shared-variable "My Computer\\MWWL Verification.lvlib\\Desired Range"(w310) -> ()  [unwired: 1 in, 1 out]
              }
              frame 14..16 {
                w311 = 20.0 ("Desired Range")
                n167 = shared-variable "My Computer\\MWWL Verification.lvlib\\Desired Range"(w311) -> ()  [unwired: 1 in, 1 out]
              }
              frame 18..22 {
                w313 = 20.0 ("Desired Range")
                # "At this point, the test is finished."
                n168 = shared-variable "My Computer\\MWWL Verification.lvlib\\Desired Range"(w313) -> ()  [unwired: 1 in, 1 out]
              }
              frame Default {
                w314 = 5.0 ("Desired Range")
                # "Default position for target."
                n169 = shared-variable "My Computer\\MWWL Verification.lvlib\\Desired Range"(w314) -> ()  [unwired: 1 in, 1 out]
              }
            }
            n170 = call "Send Set Desired Range.vi"("Desired Range"=w306, "Message Enqueuer in"=w308) -> ("Message Enqueuer out"=w307:refnum<class "Message Enqueuer.lvclass">)  [unwired: 8 in, 1 out]
          }
        }
        n171 = Select(t=Verifier_Enum."Idle" ("Verifier State"), s=w295, f=Verifier_Enum."Check Target Distance" ("Verifier State")) -> (s? t:f=w296:T1)
      }
      frame "Save to Disk" {
      }
    }
    n172 = Wait Until Next ms Multiple(millisecond multiple=u32 100) -> ()  [unwired: 1 out]
    n173 = property on="stop signal" class="Bool (strict)"() -> ("Value"=w275:bool)  [unwired: 2 in, 2 out]
    n174 = call "Elapsed Time"("Reset"=w271, "Auto Reset"=FALSE) -> ("Start Time Text"=w267:string, "Elapsed Time (s)"=w263:dbl, "Time has Elapsed"=w270:bool, "Elapsed Time Text"=w259:string)  [unwired: 10 in, 4 out]
  }
  n175 = call-parent "Actor Core.vi"("error in"=w23, "Actor in"=w19) -> ("error out"=w31:errorcluster, "Actor out"=→"Actor out":refnum<class "Actor.lvclass">)  [unwired: 8 in]
  n176 = call <vilib>:"Simple Error Handler.vi"("error in (no error)"=w31) -> ("error out"=w30:errorcluster)  [unwired: 4 in, 4 out]
  n177 = stacked-sequence {
    tunnel: [w316] -> w27
    tunnel: w30 -> [w316]
    frame #0 {
      # "Do this even if there is an error upstream."
      n178 = property on="stop signal" class="Bool (strict)"("Val(Sgnl)"=TRUE ("stop")) -> ()  [unwired: 2 in, 2 out]
    }
  }
  n179 = Unregister For Events(event registration refnum=w28, error in=w27) -> (error out=→"error out":errorcluster)
  "Time Series" <- w9
